vi "callback_send.vi"(8 "error in (no error)":errorcluster, 9 "flags":i32, 10 "buffer":u8[](array[numeric]), 11 "socket":u64) -> (0 "error out":errorcluster, 2 "bytes send":i64)   [LabVIEW 2013, in "libssh2_integration_tests.lvlib"]
doc: "Called when libssh2 wants to send data on the connection.\n\n<B>socket</B> is the socket to write to.\n<B>buffer</B> is the data to send.\n<B>flags</B> are the flags that would have been used by a send() call.\n\nReturns the number of bytes sent."
uses:
  libssh2_integration_tests.lvlib
  ws2_32.dll
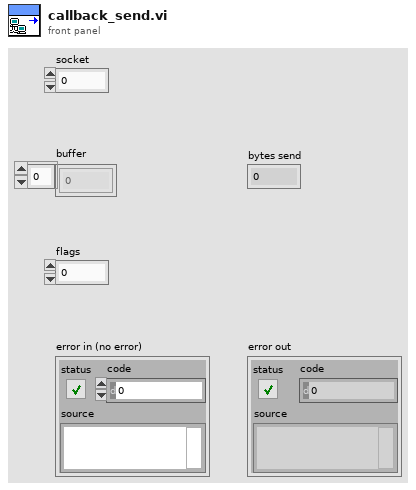
[diagram p1: front panel]
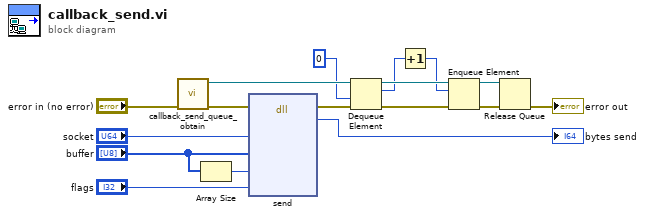
[diagram p0: block diagram]
diagram:
  n1 = call "callback_send_queue_obtain.vi"("error in (no error)"="error in (no error)") -> ("error out"=w11:errorcluster, "queue out"=w9:refnum<queue>)  [unwired: 9 in]
  n2 = Array Size(array="buffer") -> (size(s)=w16:i32)
  n3 = dll-call lib="ws2_32.dll" fn="send"(error in=w11, "s"="socket", "buf"="buffer", "len"=w16, "flags"="flags") -> (error out=w13:errorcluster, "return type"=→"bytes send":i32)  [unwired: 6 in, 1 out]
  n4 = Dequeue Element(queue=w9, timeout in ms (-1)=0, error in (no error)=w13) -> (queue out=w3:refnum<queue>, element=w2:i64, error out=w10:errorcluster)  [unwired: 1 out]
  n5 = Increment(x=w2) -> (x+1=w1:i64)
  n6 = Enqueue Element(queue=w3, element=w1, error in (no error)=w10) -> (queue out=w4:refnum<queue>, error out=w5:errorcluster)  [unwired: 1 in, 1 out]
  n7 = Release Queue(queue=w4, error in (no error)=w5) -> (error out=→"error out":errorcluster)  [unwired: 1 in, 2 out]
